vi "Array shortcut menu.vi"() -> ()   [LabVIEW 2019]
panel:
  out "Class Name":string
  in  "Tags":string[](array[string])
  in  "Stop Button":bool
  in  "Array - String":path[](array[path])
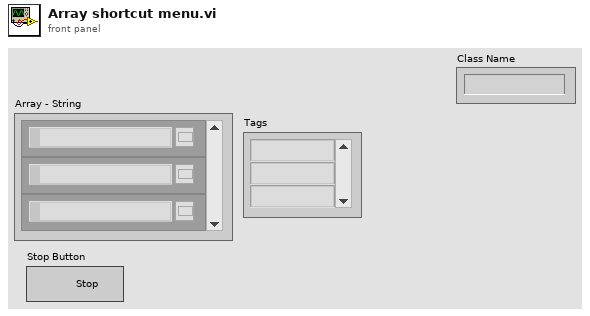
[diagram p1: front panel]
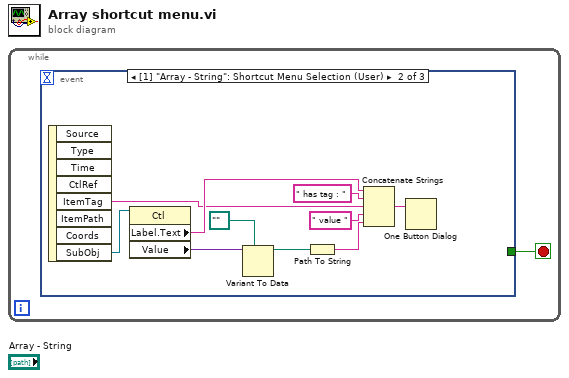
[diagram p0: block diagram]
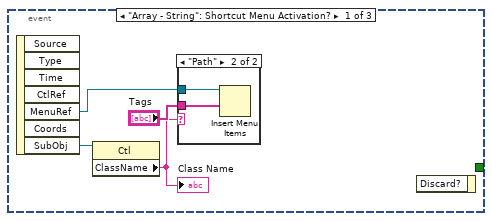
[diagram p2: hidden frame]
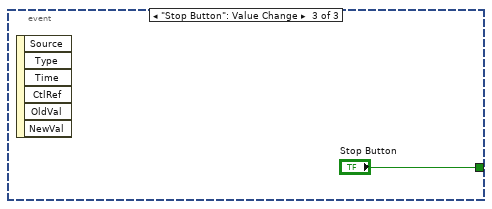
[diagram p4: hidden frame]
diagram:
  n1 = while {
    stop <- w1 stop-if-true
    n2 = event shown="[1] \"Array - String\": Shortcut Menu Selection (User)" {
      selector: _ -> [_ _ _]
      dyn-events: _ -> [_ _ _]
      timeout: _ -> [_ _ _]
      tunnel: [_ _ "Stop Button"] -> w1
      event "Array - String": Shortcut Menu Activation? {
        n3 = event-data() -> ("MenuRef"=w5:refnum<k9>, "SubObj"=w3:refnum<vi>)  [unwired: 1 in, 5 out]
        n4 = property class="Ctl"(reference=w3) -> ("ClassName"=w2:string)  [unwired: 1 in, 2 out]
        "Class Name" <- w2
        n5 = case shown="\"Path\"" w2 {
          tunnel: w5 -> [_ w7]
          tunnel: "Tags" -> [_ w6]
          frame "False", Default {
          }
          frame "Path" {
            n6 = Insert Menu Items(7:w6, 9:w7) -> ()  [unwired: 4 in, 3 out]
          }
        }
        n7 = event-data() -> ()  [unwired: 2 in, 1 out]
      }
      event "Array - String": Shortcut Menu Selection (User) {
        n8 = event-data() -> ("ItemTag"=w14:string, "SubObj"=w17:refnum<vi>)  [unwired: 1 in, 6 out]
        n9 = property class="Ctl"(reference=w17) -> ("Label.Text"=w15:string, "Value"=w13:variant)  [unwired: 1 in, 2 out]
        n10 = Variant To Data(type=path "", Variant=w13) -> (data=w11:path)  [unwired: 1 in, 1 out]
        n11 = Path To String(path=w11) -> (string=w8:string)
        n12 = Concatenate Strings(w15, " has tag : " ("string"), w14, " value " ("string"), w8) -> (w16:string)
        n13 = One Button Dialog(message=w16) -> ()  [unwired: 1 in, 1 out]
      }
      event "Stop Button": Value Change {
        n14 = event-data() -> ()  [unwired: 1 in, 6 out]
      }
    }
  }
